vi "Matlab Chirps Computation.vi"(8 "error in":errorcluster, 9 "Zoom":dbl[](array[numeric]), 10 "ROI Coordinates":T2={"XYZ Start"=[{"X"=-1.0, "Y"=-1.0, "Z"=0.0}, {"X"=-1.0, "Y"=-0.99, "Z"=0.0}, {"X"=-1.0, "Y"=-0.98, "Z"=0.0}, {"X"=-1.0, "Y"=-0.97, "Z"=0.0}, {"X"=-1.0, "Y"=-0.96, "Z"=0.0}, {"X"=-1.0, "Y"=-0.95, "Z"=0.0}, {"X"=-1.0, "Y"=-0.94, "Z"=0.0}, {"X"=-1.0, "Y"=-0.93, "Z"=0.0}, {"X"=-1.0, "Y"=-0.92, "Z"=0.0}, {"X"=-1.0, "Y"=-0.91, "Z"=0.0}, {"X"=-1.0, "Y"=-0.9, "Z"=0.0}, {"X"=-1.0, "Y"=-0.89, "Z"=0.0}, {"X"=-1.0, "Y"=-0.88, "Z"=0.0}, {"X"=-1.0, "Y"=-0.87, "Z"=0.0}, {"X"=-1.0, "Y"=-0.86, "Z"=0.0}, {"X"=-1.0, "Y"=-0.85, "Z"=0.0}, {"X"=-1.0, "Y"=-0.84, "Z"=0.0}, {"X"=-1.0, "Y"=-0.83, "Z"=0.0}, {"X"=-1.0, "Y"=-0.82, "Z"=0.0}, {"X"=-1.0, "Y"=-0.81, "Z"=0.0}, {"X"=-1.0, "Y"=-0.8, "Z"=0.0}, {"X"=-1.0, "Y"=-0.79, "Z"=0.0}, {"X"=-1.0, "Y"=-0.78, "Z"=0.0}, {"X"=-1.0, "Y"=-0.77, "Z"=0.0}, {"X"=-1.0, "Y"=-0.76, "Z"=0.0}, {"X"=-1.0, "Y"=-0.75, "Z"=0.0}, {"X"=-1.0, "Y"=-0.74, "Z"=0.0}, {"X"=-1.0, "Y"=-0.73, "Z"=0.0}, {"X"=-1.0, "Y"=-0.72, "Z"=0.0}, {"X"=-1.0, "Y"=-0.71, "Z"=0.0}, {"X"=-1.0, "Y"=-0.7, "Z"=0.0}, {"X"=-1.0, "Y"=-0.69, "Z"=0.0}, {"X"=-1.0, "Y"=-0.68, "Z"=0.0}, {"X"=-1.0, "Y"=-0.67, "Z"=0.0}, {"X"=-1.0, "Y"=-0.66, "Z"=0.0}, {"X"=-1.0, "Y"=-0.65, "Z"=0.0}, {"X"=-1.0, "Y"=-0.64, "Z"=0.0}, {"X"=-1.0, "Y"=-0.63, "Z"=0.0}, {"X"=-1.0, "Y"=-0.62, "Z"=0.0}, {"X"=-1.0, "Y"=-0.61, "Z"=0.0}, {"X"=-1.0, "Y"=-0.6, "Z"=0.0}, {"X"=-1.0, "Y"=-0.59, "Z"=0.0}, {"X"=-1.0, "Y"=-0.58, "Z"=0.0}, {"X"=-1.0, "Y"=-0.57, "Z"=0.0}, {"X"=-1.0, "Y"=-0.56, "Z"=0.0}, {"X"=-1.0, "Y"=-0.55, "Z"=0.0}, {"X"=-1.0, "Y"=-0.54, "Z"=0.0}, {"X"=-1.0, "Y"=-0.53, "Z"=0.0}, {"X"=-1.0, "Y"=-0.52, "Z"=0.0}, {"X"=-1.0, "Y"=-0.51, "Z"=0.0}, {"X"=-1.0, "Y"=-0.5, "Z"=0.0}, {"X"=-1.0, "Y"=-0.49, "Z"=0.0}, {"X"=-1.0, "Y"=-0.48, "Z"=0.0}, {"X"=-1.0, "Y"=-0.47, "Z"=0.0}, {"X"=-1.0, "Y"=-0.46, "Z"=0.0}, {"X"=-1.0, "Y"=-0.45, "Z"=0.0}, {"X"=-1.0, "Y"=-0.44, "Z"=0.0}, {"X"=-1.0, "Y"=-0.43, "Z"=0.0}, {"X"=-1.0, "Y"=-0.42, "Z"=0.0}, {"X"=-1.0, "Y"=-0.41, "Z"=0.0}, {"X"=-1.0, "Y"=-0.4, "Z"=0.0}, {"X"=-1.0, "Y"=-0.39, "Z"=0.0}, {"X"=-1.0, "Y"=-0.38, "Z"=0.0}, {"X"=-1.0, "Y"=-0.37, "Z"=0.0}, {"X"=-1.0, "Y"=-0.36, "Z"=0.0}, {"X"=-1.0, "Y"=-0.35, "Z"=0.0}, {"X"=-1.0, "Y"=-0.34, "Z"=0.0}, {"X"=-1.0, "Y"=-0.33, "Z"=0.0}, {"X"=-1.0, "Y"=-0.32, "Z"=0.0}, {"X"=-1.0, "Y"=-0.31, "Z"=0.0}, {"X"=-1.0, "Y"=-0.3, "Z"=0.0}, {"X"=-1.0, "Y"=-0.29, "Z"=0.0}, {"X"=-1.0, "Y"=-0.28, "Z"=0.0}, {"X"=-1.0, "Y"=-0.27, "Z"=0.0}, {"X"=-1.0, "Y"=-0.26, "Z"=0.0}, {"X"=-1.0, "Y"=-0.25, "Z"=0.0}, {"X"=-1.0, "Y"=-0.24, "Z"=0.0}, {"X"=-1.0, "Y"=-0.23, "Z"=0.0}, {"X"=-1.0, "Y"=-0.22, "Z"=0.0}, {"X"=-1.0, "Y"=-0.21, "Z"=0.0}, {"X"=-1.0, "Y"=-0.2, "Z"=0.0}, {"X"=-1.0, "Y"=-0.19, "Z"=0.0}, {"X"=-1.0, "Y"=-0.18, "Z"=0.0}, {"X"=-1.0, "Y"=-0.17, "Z"=0.0}, {"X"=-1.0, "Y"=-0.16, "Z"=0.0}, {"X"=-1.0, "Y"=-0.15, "Z"=0.0}, {"X"=-1.0, "Y"=-0.14, "Z"=0.0}, {"X"=-1.0, "Y"=-0.13, "Z"=0.0}, {"X"=-1.0, "Y"=-0.12, "Z"=0.0}, {"X"=-1.0, "Y"=-0.11, "Z"=0.0}, {"X"=-1.0, "Y"=-0.1, "Z"=0.0}, {"X"=-1.0, "Y"=-0.09, "Z"=0.0}, {"X"=-1.0, "Y"=-0.08, "Z"=0.0}, {"X"=-1.0, "Y"=-0.07, "Z"=0.0}, {"X"=-1.0, "Y"=-0.06, "Z"=0.0}, {"X"=-1.0, "Y"=-0.05, "Z"=0.0}, {"X"=-1.0, "Y"=-0.04, "Z"=0.0}, {"X"=-1.0, "Y"=-0.03, "Z"=0.0}, {"X"=-1.0, "Y"=-0.02, "Z"=0.0}, {"X"=-1.0, "Y"=-0.01, "Z"=0.0}, {"X"=-1.0, "Y"=0.0, "Z"=0.0}, {"X"=-1.0, "Y"=0.01, "Z"=0.0}, {"X"=-1.0, "Y"=0.02, "Z"=0.0}, {"X"=-1.0, "Y"=0.03, "Z"=0.0}, {"X"=-1.0, "Y"=0.04, "Z"=0.0}, {"X"=-1.0, "Y"=0.05, "Z"=0.0}, {"X"=-1.0, "Y"=0.06, "Z"=0.0}, {"X"=-1.0, "Y"=0.07, "Z"=0.0}, {"X"=-1.0, "Y"=0.08, "Z"=0.0}, {"X"=-1.0, "Y"=0.09, "Z"=0.0}, {"X"=-1.0, "Y"=0.1, "Z"=0.0}, {"X"=-1.0, "Y"=0.11, "Z"=0.0}, {"X"=-1.0, "Y"=0.12, "Z"=0.0}, {"X"=-1.0, "Y"=0.13, "Z"=0.0}, {"X"=-1.0, "Y"=0.14, "Z"=0.0}, {"X"=-1.0, "Y"=0.15, "Z"=0.0}, {"X"=-1.0, "Y"=0.16, "Z"=0.0}, {"X"=-1.0, "Y"=0.17, "Z"=0.0}, {"X"=-1.0, "Y"=0.18, "Z"=0.0}, {"X"=-1.0, "Y"=0.19, "Z"=0.0}, {"X"=-1.0, "Y"=0.2, "Z"=0.0}, {"X"=-1.0, "Y"=0.21, "Z"=0.0}, {"X"=-1.0, "Y"=0.22, "Z"=0.0}, {"X"=-1.0, "Y"=0.23, "Z"=0.0}, {"X"=-1.0, "Y"=0.24, "Z"=0.0}, {"X"=-1.0, "Y"=0.25, "Z"=0.0}, {"X"=-1.0, "Y"=0.26, "Z"=0.0}, {"X"=-1.0, "Y"=0.27, "Z"=0.0}, {"X"=-1.0, "Y"=0.28, "Z"=0.0}, {"X"=-1.0, "Y"=0.29, "Z"=0.0}, {"X"=-1.0, "Y"=0.3, "Z"=0.0}, {"X"=-1.0, "Y"=0.31, "Z"=0.0}, {"X"=-1.0, "Y"=0.32, "Z"=0.0}, {"X"=-1.0, "Y"=0.33, "Z"=0.0}, {"X"=-1.0, "Y"=0.34, "Z"=0.0}, {"X"=-1.0, "Y"=0.35, "Z"=0.0}, {"X"=-1.0, "Y"=0.36, "Z"=0.0}, {"X"=-1.0, "Y"=0.37, "Z"=0.0}, {"X"=-1.0, "Y"=0.38, "Z"=0.0}, {"X"=-1.0, "Y"=0.39, "Z"=0.0}, {"X"=-1.0, "Y"=0.4, "Z"=0.0}, {"X"=-1.0, "Y"=0.41, "Z"=0.0}, {"X"=-1.0, "Y"=0.42, "Z"=0.0}, {"X"=-1.0, "Y"=0.43, "Z"=0.0}, {"X"=-1.0, "Y"=0.44, "Z"=0.0}, {"X"=-1.0, "Y"=0.45, "Z"=0.0}, {"X"=-1.0, "Y"=0.46, "Z"=0.0}, {"X"=-1.0, "Y"=0.47, "Z"=0.0}, {"X"=-1.0, "Y"=0.48, "Z"=0.0}, {"X"=-1.0, "Y"=0.49, "Z"=0.0}, {"X"=-1.0, "Y"=0.5, "Z"=0.0}, {"X"=-1.0, "Y"=0.51, "Z"=0.0}, {"X"=-1.0, "Y"=0.52, "Z"=0.0}, {"X"=-1.0, "Y"=0.53, "Z"=0.0}, {"X"=-1.0, "Y"=0.54, "Z"=0.0}, {"X"=-1.0, "Y"=0.55, "Z"=0.0}, {"X"=-1.0, "Y"=0.56, "Z"=0.0}, {"X"=-1.0, "Y"=0.57, "Z"=0.0}, {"X"=-1.0, "Y"=0.58, "Z"=0.0}, {"X"=-1.0, "Y"=0.59, "Z"=0.0}, {"X"=-1.0, "Y"=0.6, "Z"=0.0}, {"X"=-1.0, "Y"=0.61, "Z"=0.0}, {"X"=-1.0, "Y"=0.62, "Z"=0.0}, {"X"=-1.0, "Y"=0.63, "Z"=0.0}, {"X"=-1.0, "Y"=0.64, "Z"=0.0}, {"X"=-1.0, "Y"=0.65, "Z"=0.0}, {"X"=-1.0, "Y"=0.66, "Z"=0.0}, {"X"=-1.0, "Y"=0.67, "Z"=0.0}, {"X"=-1.0, "Y"=0.68, "Z"=0.0}, {"X"=-1.0, "Y"=0.69, "Z"=0.0}, {"X"=-1.0, "Y"=0.7, "Z"=0.0}, {"X"=-1.0, "Y"=0.71, "Z"=0.0}, {"X"=-1.0, "Y"=0.72, "Z"=0.0}, {"X"=-1.0, "Y"=0.73, "Z"=0.0}, {"X"=-1.0, "Y"=0.74, "Z"=0.0}, {"X"=-1.0, "Y"=0.75, "Z"=0.0}, {"X"=-1.0, "Y"=0.76, "Z"=0.0}, {"X"=-1.0, "Y"=0.77, "Z"=0.0}, {"X"=-1.0, "Y"=0.78, "Z"=0.0}, {"X"=-1.0, "Y"=0.79, "Z"=0.0}, {"X"=-1.0, "Y"=0.8, "Z"=0.0}, {"X"=-1.0, "Y"=0.81, "Z"=0.0}, {"X"=-1.0, "Y"=0.82, "Z"=0.0}, {"X"=-1.0, "Y"=0.83, "Z"=0.0}, {"X"=-1.0, "Y"=0.84, "Z"=0.0}, {"X"=-1.0, "Y"=0.85, "Z"=0.0}, {"X"=-1.0, "Y"=0.86, "Z"=0.0}, {"X"=-1.0, "Y"=0.87, "Z"=0.0}, {"X"=-1.0, "Y"=0.88, "Z"=0.0}, {"X"=-1.0, "Y"=0.89, "Z"=0.0}, {"X"=-1.0, "Y"=0.9, "Z"=0.0}, {"X"=-1.0, "Y"=0.91, "Z"=0.0}, {"X"=-1.0, "Y"=0.92, "Z"=0.0}, {"X"=-1.0, "Y"=0.93, "Z"=0.0}, {"X"=-1.0, "Y"=0.94, "Z"=0.0}, {"X"=-1.0, "Y"=0.95, "Z"=0.0}, {"X"=-1.0, "Y"=0.96, "Z"=0.0}, {"X"=-1.0, "Y"=0.97, "Z"=0.0}, {"X"=-1.0, "Y"=0.98, "Z"=0.0}, {"X"=-1.0, "Y"=0.99, "Z"=0.0}], "XYZ Stop"=[{"X"=1.0, "Y"=-1.0, "Z"=0.0}, {"X"=1.0, "Y"=-0.99, "Z"=0.0}, {"X"=1.0, "Y"=-0.98, "Z"=0.0}, {"X"=1.0, "Y"=-0.97, "Z"=0.0}, {"X"=1.0, "Y"=-0.96, "Z"=0.0}, {"X"=1.0, "Y"=-0.95, "Z"=0.0}, {"X"=1.0, "Y"=-0.94, "Z"=0.0}, {"X"=1.0, "Y"=-0.93, "Z"=0.0}, {"X"=1.0, "Y"=-0.92, "Z"=0.0}, {"X"=1.0, "Y"=-0.91, "Z"=0.0}, {"X"=1.0, "Y"=-0.9, "Z"=0.0}, {"X"=1.0, "Y"=-0.89, "Z"=0.0}, {"X"=1.0, "Y"=-0.88, "Z"=0.0}, {"X"=1.0, "Y"=-0.87, "Z"=0.0}, {"X"=1.0, "Y"=-0.86, "Z"=0.0}, {"X"=1.0, "Y"=-0.85, "Z"=0.0}, {"X"=1.0, "Y"=-0.84, "Z"=0.0}, {"X"=1.0, "Y"=-0.83, "Z"=0.0}, {"X"=1.0, "Y"=-0.82, "Z"=0.0}, {"X"=1.0, "Y"=-0.81, "Z"=0.0}, {"X"=1.0, "Y"=-0.8, "Z"=0.0}, {"X"=1.0, "Y"=-0.79, "Z"=0.0}, {"X"=1.0, "Y"=-0.78, "Z"=0.0}, {"X"=1.0, "Y"=-0.77, "Z"=0.0}, {"X"=1.0, "Y"=-0.76, "Z"=0.0}, {"X"=1.0, "Y"=-0.75, "Z"=0.0}, {"X"=1.0, "Y"=-0.74, "Z"=0.0}, {"X"=1.0, "Y"=-0.73, "Z"=0.0}, {"X"=1.0, "Y"=-0.72, "Z"=0.0}, {"X"=1.0, "Y"=-0.71, "Z"=0.0}, {"X"=1.0, "Y"=-0.7, "Z"=0.0}, {"X"=1.0, "Y"=-0.69, "Z"=0.0}, {"X"=1.0, "Y"=-0.68, "Z"=0.0}, {"X"=1.0, "Y"=-0.67, "Z"=0.0}, {"X"=1.0, "Y"=-0.66, "Z"=0.0}, {"X"=1.0, "Y"=-0.65, "Z"=0.0}, {"X"=1.0, "Y"=-0.64, "Z"=0.0}, {"X"=1.0, "Y"=-0.63, "Z"=0.0}, {"X"=1.0, "Y"=-0.62, "Z"=0.0}, {"X"=1.0, "Y"=-0.61, "Z"=0.0}, {"X"=1.0, "Y"=-0.6, "Z"=0.0}, {"X"=1.0, "Y"=-0.59, "Z"=0.0}, {"X"=1.0, "Y"=-0.58, "Z"=0.0}, {"X"=1.0, "Y"=-0.57, "Z"=0.0}, {"X"=1.0, "Y"=-0.56, "Z"=0.0}, {"X"=1.0, "Y"=-0.55, "Z"=0.0}, {"X"=1.0, "Y"=-0.54, "Z"=0.0}, {"X"=1.0, "Y"=-0.53, "Z"=0.0}, {"X"=1.0, "Y"=-0.52, "Z"=0.0}, {"X"=1.0, "Y"=-0.51, "Z"=0.0}, {"X"=1.0, "Y"=-0.5, "Z"=0.0}, {"X"=1.0, "Y"=-0.49, "Z"=0.0}, {"X"=1.0, "Y"=-0.48, "Z"=0.0}, {"X"=1.0, "Y"=-0.47, "Z"=0.0}, {"X"=1.0, "Y"=-0.46, "Z"=0.0}, {"X"=1.0, "Y"=-0.45, "Z"=0.0}, {"X"=1.0, "Y"=-0.44, "Z"=0.0}, {"X"=1.0, "Y"=-0.43, "Z"=0.0}, {"X"=1.0, "Y"=-0.42, "Z"=0.0}, {"X"=1.0, "Y"=-0.41, "Z"=0.0}, {"X"=1.0, "Y"=-0.4, "Z"=0.0}, {"X"=1.0, "Y"=-0.39, "Z"=0.0}, {"X"=1.0, "Y"=-0.38, "Z"=0.0}, {"X"=1.0, "Y"=-0.37, "Z"=0.0}, {"X"=1.0, "Y"=-0.36, "Z"=0.0}, {"X"=1.0, "Y"=-0.35, "Z"=0.0}, {"X"=1.0, "Y"=-0.34, "Z"=0.0}, {"X"=1.0, "Y"=-0.33, "Z"=0.0}, {"X"=1.0, "Y"=-0.32, "Z"=0.0}, {"X"=1.0, "Y"=-0.31, "Z"=0.0}, {"X"=1.0, "Y"=-0.3, "Z"=0.0}, {"X"=1.0, "Y"=-0.29, "Z"=0.0}, {"X"=1.0, "Y"=-0.28, "Z"=0.0}, {"X"=1.0, "Y"=-0.27, "Z"=0.0}, {"X"=1.0, "Y"=-0.26, "Z"=0.0}, {"X"=1.0, "Y"=-0.25, "Z"=0.0}, {"X"=1.0, "Y"=-0.24, "Z"=0.0}, {"X"=1.0, "Y"=-0.23, "Z"=0.0}, {"X"=1.0, "Y"=-0.22, "Z"=0.0}, {"X"=1.0, "Y"=-0.21, "Z"=0.0}, {"X"=1.0, "Y"=-0.2, "Z"=0.0}, {"X"=1.0, "Y"=-0.19, "Z"=0.0}, {"X"=1.0, "Y"=-0.18, "Z"=0.0}, {"X"=1.0, "Y"=-0.17, "Z"=0.0}, {"X"=1.0, "Y"=-0.16, "Z"=0.0}, {"X"=1.0, "Y"=-0.15, "Z"=0.0}, {"X"=1.0, "Y"=-0.14, "Z"=0.0}, {"X"=1.0, "Y"=-0.13, "Z"=0.0}, {"X"=1.0, "Y"=-0.12, "Z"=0.0}, {"X"=1.0, "Y"=-0.11, "Z"=0.0}, {"X"=1.0, "Y"=-0.1, "Z"=0.0}, {"X"=1.0, "Y"=-0.09, "Z"=0.0}, {"X"=1.0, "Y"=-0.08, "Z"=0.0}, {"X"=1.0, "Y"=-0.07, "Z"=0.0}, {"X"=1.0, "Y"=-0.06, "Z"=0.0}, {"X"=1.0, "Y"=-0.05, "Z"=0.0}, {"X"=1.0, "Y"=-0.04, "Z"=0.0}, {"X"=1.0, "Y"=-0.03, "Z"=0.0}, {"X"=1.0, "Y"=-0.02, "Z"=0.0}, {"X"=1.0, "Y"=-0.01, "Z"=0.0}, {"X"=1.0, "Y"=0.0, "Z"=0.0}, {"X"=1.0, "Y"=0.01, "Z"=0.0}, {"X"=1.0, "Y"=0.02, "Z"=0.0}, {"X"=1.0, "Y"=0.03, "Z"=0.0}, {"X"=1.0, "Y"=0.04, "Z"=0.0}, {"X"=1.0, "Y"=0.05, "Z"=0.0}, {"X"=1.0, "Y"=0.06, "Z"=0.0}, {"X"=1.0, "Y"=0.07, "Z"=0.0}, {"X"=1.0, "Y"=0.08, "Z"=0.0}, {"X"=1.0, "Y"=0.09, "Z"=0.0}, {"X"=1.0, "Y"=0.1, "Z"=0.0}, {"X"=1.0, "Y"=0.11, "Z"=0.0}, {"X"=1.0, "Y"=0.12, "Z"=0.0}, {"X"=1.0, "Y"=0.13, "Z"=0.0}, {"X"=1.0, "Y"=0.14, "Z"=0.0}, {"X"=1.0, "Y"=0.15, "Z"=0.0}, {"X"=1.0, "Y"=0.16, "Z"=0.0}, {"X"=1.0, "Y"=0.17, "Z"=0.0}, {"X"=1.0, "Y"=0.18, "Z"=0.0}, {"X"=1.0, "Y"=0.19, "Z"=0.0}, {"X"=1.0, "Y"=0.2, "Z"=0.0}, {"X"=1.0, "Y"=0.21, "Z"=0.0}, {"X"=1.0, "Y"=0.22, "Z"=0.0}, {"X"=1.0, "Y"=0.23, "Z"=0.0}, {"X"=1.0, "Y"=0.24, "Z"=0.0}, {"X"=1.0, "Y"=0.25, "Z"=0.0}, {"X"=1.0, "Y"=0.26, "Z"=0.0}, {"X"=1.0, "Y"=0.27, "Z"=0.0}, {"X"=1.0, "Y"=0.28, "Z"=0.0}, {"X"=1.0, "Y"=0.29, "Z"=0.0}, {"X"=1.0, "Y"=0.3, "Z"=0.0}, {"X"=1.0, "Y"=0.31, "Z"=0.0}, {"X"=1.0, "Y"=0.32, "Z"=0.0}, {"X"=1.0, "Y"=0.33, "Z"=0.0}, {"X"=1.0, "Y"=0.34, "Z"=0.0}, {"X"=1.0, "Y"=0.35, "Z"=0.0}, {"X"=1.0, "Y"=0.36, "Z"=0.0}, {"X"=1.0, "Y"=0.37, "Z"=0.0}, {"X"=1.0, "Y"=0.38, "Z"=0.0}, {"X"=1.0, "Y"=0.39, "Z"=0.0}, {"X"=1.0, "Y"=0.4, "Z"=0.0}, {"X"=1.0, "Y"=0.41, "Z"=0.0}, {"X"=1.0, "Y"=0.42, "Z"=0.0}, {"X"=1.0, "Y"=0.43, "Z"=0.0}, {"X"=1.0, "Y"=0.44, "Z"=0.0}, {"X"=1.0, "Y"=0.45, "Z"=0.0}, {"X"=1.0, "Y"=0.46, "Z"=0.0}, {"X"=1.0, "Y"=0.47, "Z"=0.0}, {"X"=1.0, "Y"=0.48, "Z"=0.0}, {"X"=1.0, "Y"=0.49, "Z"=0.0}, {"X"=1.0, "Y"=0.5, "Z"=0.0}, {"X"=1.0, "Y"=0.51, "Z"=0.0}, {"X"=1.0, "Y"=0.52, "Z"=0.0}, {"X"=1.0, "Y"=0.53, "Z"=0.0}, {"X"=1.0, "Y"=0.54, "Z"=0.0}, {"X"=1.0, "Y"=0.55, "Z"=0.0}, {"X"=1.0, "Y"=0.56, "Z"=0.0}, {"X"=1.0, "Y"=0.57, "Z"=0.0}, {"X"=1.0, "Y"=0.58, "Z"=0.0}, {"X"=1.0, "Y"=0.59, "Z"=0.0}, {"X"=1.0, "Y"=0.6, "Z"=0.0}, {"X"=1.0, "Y"=0.61, "Z"=0.0}, {"X"=1.0, "Y"=0.62, "Z"=0.0}, {"X"=1.0, "Y"=0.63, "Z"=0.0}, {"X"=1.0, "Y"=0.64, "Z"=0.0}, {"X"=1.0, "Y"=0.65, "Z"=0.0}, {"X"=1.0, "Y"=0.66, "Z"=0.0}, {"X"=1.0, "Y"=0.67, "Z"=0.0}, {"X"=1.0, "Y"=0.68, "Z"=0.0}, {"X"=1.0, "Y"=0.69, "Z"=0.0}, {"X"=1.0, "Y"=0.7, "Z"=0.0}, {"X"=1.0, "Y"=0.71, "Z"=0.0}, {"X"=1.0, "Y"=0.72, "Z"=0.0}, {"X"=1.0, "Y"=0.73, "Z"=0.0}, {"X"=1.0, "Y"=0.74, "Z"=0.0}, {"X"=1.0, "Y"=0.75, "Z"=0.0}, {"X"=1.0, "Y"=0.76, "Z"=0.0}, {"X"=1.0, "Y"=0.77, "Z"=0.0}, {"X"=1.0, "Y"=0.78, "Z"=0.0}, {"X"=1.0, "Y"=0.79, "Z"=0.0}, {"X"=1.0, "Y"=0.8, "Z"=0.0}, {"X"=1.0, "Y"=0.81, "Z"=0.0}, {"X"=1.0, "Y"=0.82, "Z"=0.0}, {"X"=1.0, "Y"=0.83, "Z"=0.0}, {"X"=1.0, "Y"=0.84, "Z"=0.0}, {"X"=1.0, "Y"=0.85, "Z"=0.0}, {"X"=1.0, "Y"=0.86, "Z"=0.0}, {"X"=1.0, "Y"=0.87, "Z"=0.0}, {"X"=1.0, "Y"=0.88, "Z"=0.0}, {"X"=1.0, "Y"=0.89, "Z"=0.0}, {"X"=1.0, "Y"=0.9, "Z"=0.0}, {"X"=1.0, "Y"=0.91, "Z"=0.0}, {"X"=1.0, "Y"=0.92, "Z"=0.0}, {"X"=1.0, "Y"=0.93, "Z"=0.0}, {"X"=1.0, "Y"=0.94, "Z"=0.0}, {"X"=1.0, "Y"=0.95, "Z"=0.0}, {"X"=1.0, "Y"=0.96, "Z"=0.0}, {"X"=1.0, "Y"=0.97, "Z"=0.0}, {"X"=1.0, "Y"=0.98, "Z"=0.0}, {"X"=1.0, "Y"=0.99, "Z"=0.0}]}, 11 "AOL_Globals":T3={"Imaging Protocol"=enum."Live Imaging", "Number of POI"=0, "Number of Miniscans"=0, "Number of Trials"=1, "Number of Cycles "=0, "# Averaged Frames"=1, "Laser power (%)"=7, "Pockels"=0.0, "Acquisition Length (sec)"=0.0, "Fill time (us)"=24.5, "POI Dwell time (us)"=4.0, "Miniscan Dwell time per pixel (us)"=0.0, "PMT 1"=500.0, "PMT 2"=500.0, "Back Apperture"=0.0, "Frame Size"=200, "Center Frequency"=36.28048780487805, "Field of View"=4.349999904632568, "DwellTime (us)"=0.1, "Wavelength (nm)"=820.0, "Zoom"=1.0, "AOL Z"=0.0, "AOL Mode"=enum."Raster", "GridXY"=0.0, "GridZ"=0.0, "TriggerPeriod (sec)"=0.0, "Number of Pixels in Miniscan"=0, "Experiment folder path"=path "", "X centre"=0.0, "Y centre"=0.0, "Angle (degrees)"=0.0, "Plane Mode"=0, "Threshold"=[], "Regenerate Chirps"=FALSE, "Rectangle ROI length (pixels)"=0, "Rectangle ROI height (pixels)"=0, "AOD fill"=0, "Samples Wait after Trigger"=0, "StartUp Delay"=0, "Slip Cycle"=163840, "Add Cycle"=FALSE} {"Plane Mode" items=["XY Plane"]; "Frame Size" items=["100X100"=100, "128X128"=128, "200X200"=200, "256X256"=256, "512X512"=512, "1024x1024"=1024, "2048x2048"=2048]; "Back Apperture" format="%#.6g"; "Pockels" format="%#.6g"; "PMT 2" format="%#.6g"; "PMT 1" format="%#.6g"; "Angle (degrees)" format="%#.6g"; "POI Dwell time (us)" format="%#.6g"}) -> (0 "error out":errorcluster, 1 "systemVariables":dbl[](array[numeric]), 2 "scanVariables":dbl[][](array[numeric]), 3 "Chirp Parameters":T1)   [LabVIEW 2013]
uses:
  Typedefs/Controls/AOL_Globals.ctl
  Typedefs/Imaging Protocols enum.ctl
  Typedefs/Frame Size.ctl
  Typedefs/AOL modes.ctl
  Typedefs/Plane Mode.ctl
panel:
  out "Execution time (ms)":u32
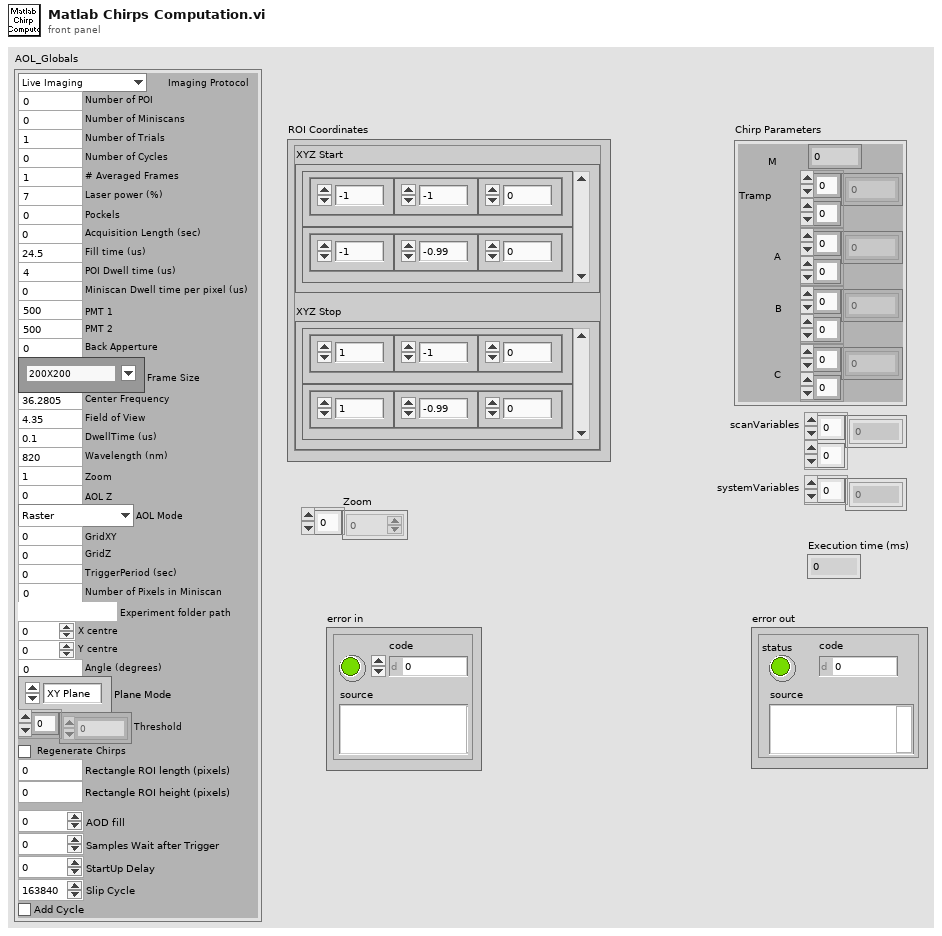
[diagram p1: front panel]
types:
  T1 = cluster{"M ":dbl, "Tramp":dbl[][], "A":dbl[][], "B":dbl[][], "C":dbl[][]}
  T2 = cluster{"XYZ Start":cluster{"X":sgl, "Y":sgl, "Z":sgl}[], "XYZ Stop":cluster{"X":sgl, "Y":sgl, "Z":sgl}[]}
  T3 = typedef "AOL_Globals.ctl" = cluster{"Imaging Protocol":T4, "Number of POI":u16, "Number of Miniscans":u16, "Number of Trials":u16, "Number of Cycles ":u64, "# Averaged Frames":u16, "Laser power (%)":u8, "Pockels":dbl, "Acquisition Length (sec)":dbl, "Fill time (us)":dbl, "POI Dwell time (us)":dbl, "Miniscan Dwell time per pixel (us)":dbl, "PMT 1":dbl, "PMT 2":dbl, "Back Apperture":dbl, "Frame Size":T5, "Center Frequency":dbl, "Field of View":dbl, "DwellTime (us)":dbl, "Wavelength (nm)":dbl, "Zoom":dbl, "AOL Z":dbl, "AOL Mode":T6, "GridXY":dbl, "GridZ":dbl, "TriggerPeriod (sec)":dbl, "Number of Pixels in Miniscan":u16, "Experiment folder path":path, "X centre":dbl, "Y centre":dbl, "Angle (degrees)":dbl, "Plane Mode":T7, "Threshold":u16[], "Regenerate Chirps":bool, "Rectangle ROI length (pixels)":u16, "Rectangle ROI height (pixels)":u16, "AOD fill":u16, "Samples Wait after Trigger":u16, "StartUp Delay":i32, "Slip Cycle":u32, "Add Cycle":bool}
  T4 = typedef "Imaging Protocols enum.ctl" = enum16{"AOL Z-Stack", "Motor Z Stack", "Functional Acquisition", "Single Plane Acquisition", "Volume Acquisition", "Live Imaging", "Live Plane Imaging", "Live Volume Imaging"}
  T5 = typedef "Frame Size.ctl" = u16
  T6 = typedef "AOL modes.ctl" = enum16{"Raster", "Structural", "Pointing", "Mini Scan", "Alignment"}
  T7 = typedef "Plane Mode.ctl" = u16
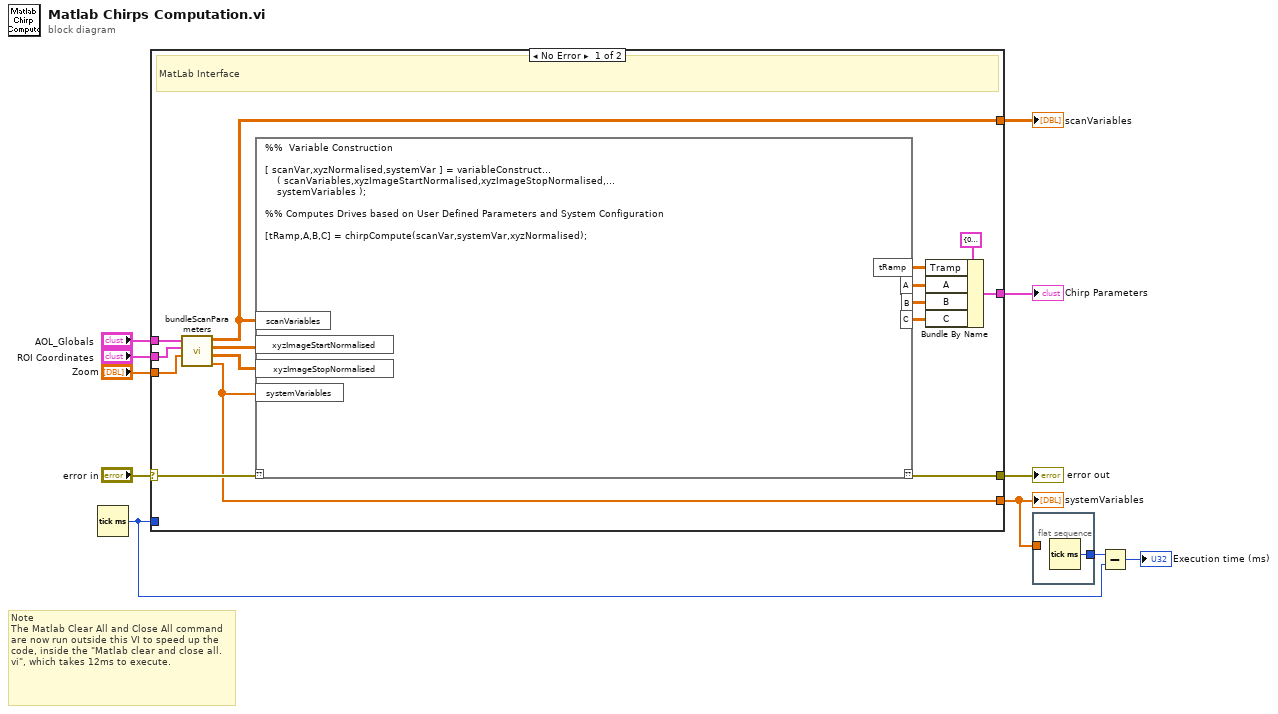
[diagram p0: block diagram]
diagram:
  # "Note\nThe Matlab Clear All and Close All command are now run outside this VI to speed up the code, inside the \"Matlab clear and close all.vi\", which takes 12ms to execute."
  n1 = Tick Count (ms)() -> (millisecond timer value=w6:u32)
  n2 = case shown="No Error" "error in" {
    selector: "error in" -> [w26 w27]
    tunnel: [w25 w27] -> w9
    tunnel: "ROI Coordinates" -> [w23 _]
    tunnel: "AOL_Globals" -> [w24 _]
    tunnel: [w19 _] -> w2
    tunnel: [w14 _] -> w3
    tunnel: [w13 _] -> w4
    tunnel: "Zoom" -> [w12 _]
    tunnel: w6 -> [_ _]
    frame No Error {
      # "MatLab Interface"
      n3 = call "bundleScanParameters.vi"("Zoom"=w12, "xyzNormalizedCoordinates"=w23, "AOL_Globals"=w24) -> ("systemVariables"=w14:dbl[], "xyzImageStopNormalised"=w21:dbl[][], "xyzImageStartNormalised"=w22:dbl[][], "scanVariables"=w13:dbl[][])  [unwired: 5 in]
      n4 = script code="%%  Variable Construction\n\n[ scanVar,xyzNormalised,systemVar ] = variableConstruct...\n    ( scanVariables,xyzImageStartNormalised,xyzImageStopNormalised,...\n    systemVariables );\n\n%% Computes Drives based on User Defined Parameters and System Configuration\n\n[tRamp,A,B,C] = chirpCompute(scanVar,systemVar,xyzNormalised);"("??"=w26, "scanVariables"=w13, "xyzImageStartNormalised"=w22, "xyzImageStopNormalised"=w21, "systemVariables"=w14) -> ("??"=w25:errorcluster, "tRamp"=w15:dbl[][], "A"=w16:dbl[][], "B"=w17:dbl[][], "C"=w18:dbl[][])
      n5 = Bundle By Name(cluster=T1 {"M "=0.0, "Tramp"=[], "A"=[], "B"=[], "C"=[]} ("Chirp Parametesr"), "Tramp"=w15, "A"=w16, "B"=w17, "C"=w18) -> (w19:T1)
    }
    frame Error {
    }
  }
  "error out" <- w9
  "Chirp Parameters" <- w2
  "systemVariables" <- w3
  "scanVariables" <- w4
  n6 = flat-sequence {
    tunnel: w3 -> [_]
    tunnel: [w28] -> w7
    frame #0 {
      n7 = Tick Count (ms)() -> (millisecond timer value=w28:u32)
    }
  }
  n8 = Subtract(x=w7, y=w6) -> (x-y=→"Execution time (ms)":u32)
